vi "(SubVI)I2C_Log.vi"(5 "Data Size":T2, 7 "R/W":T1, 8 "error in (no error)":errorcluster caption="에러 입력(에러 없음)", 9 "Data":u16 format="%.0x", 10 "Address":u16 format="%.0x", 11 "Log Ref":refnum<vi>) -> (0 "error out":errorcluster caption="에러 출력", 3 "Log":string)   [LabVIEW 2020]
uses:
  Controls/(Ctrl)I2C_Data Size.ctl
  Controls/(Ctrl)I2C_RW.ctl
panel:
  # "(SubVI)I2C_Log.vi By hspark\n\nDescription : I2C 통신 결과 Log 문자열을 생성하고 Log 문자열 인디케이터 참조를 연결한 경우 Log를 업데이트 하는VI\n\nInput : \n1. Log Ref : 업데이트할 Log 문자열 인디케이터의 참조. 입력하지 않는 경우 Log 문자열만 출력하고, 인디케이터 업데이트는 무시됨\n2. Address : 생성할 Log의 Address 부분\n3. Data : 생성할 Log의 Data 부분\n4. R/W : Read/Write 구분\n5. Data Size : 생성할 Log의 비트 크기\n\nOutput : \n1. Log : 생성된 Log 문자열 출력\n\nLabVIEW Version : 2020 SP1 이상\n\nNote : 에러 발생 시 에러 종류를 Log로 출력함. \n\nUpdate : 2021.10.06"
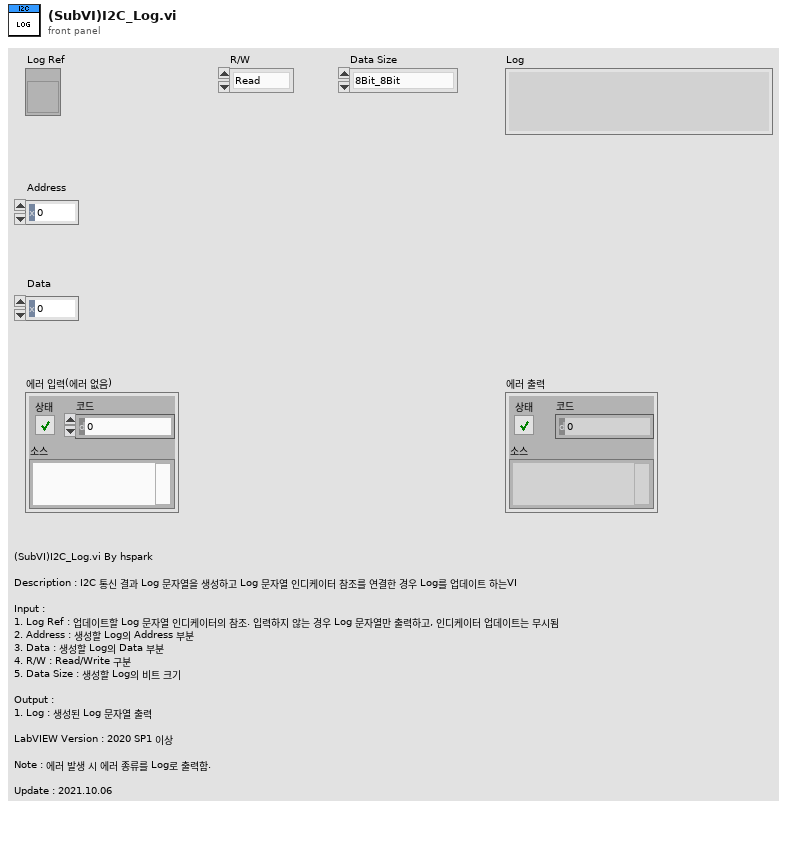
[diagram p1: front panel]
types:
  T1 = typedef "(Ctrl)I2C_RW.ctl" = enum16{"Read", "Write"}
  T2 = typedef "(Ctrl)I2C_Data Size.ctl" = enum16{"8Bit_8Bit", "16Bit_16Bit", "16Bit_8Bit"}
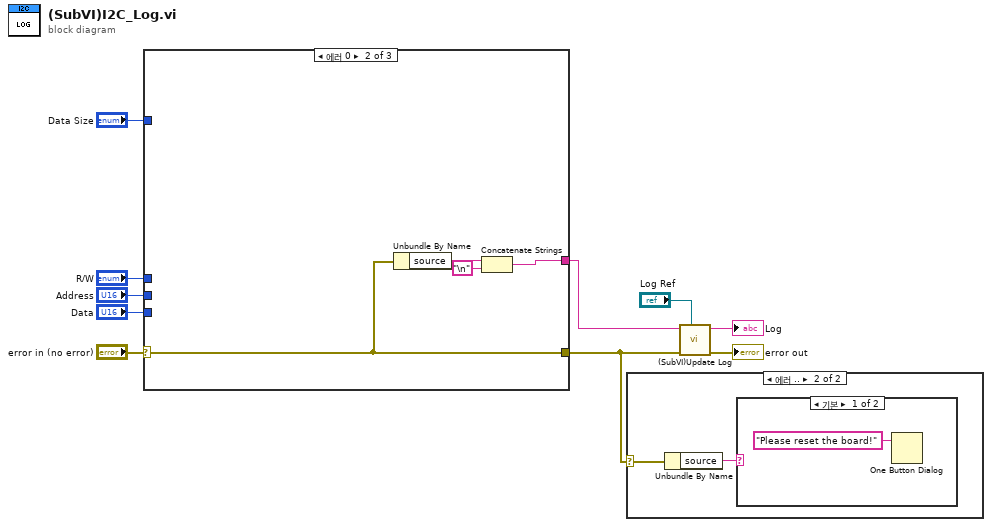
[diagram p0: block diagram]
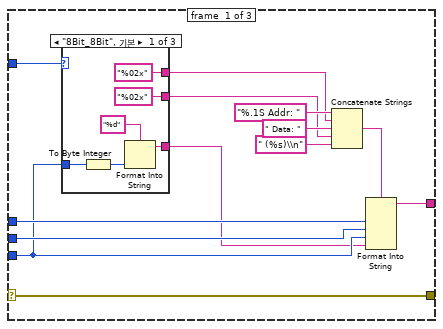
[diagram p4: hidden frame]
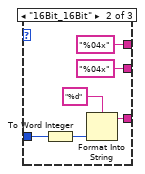
[diagram p5: hidden frame]
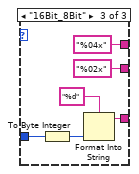
[diagram p6: hidden frame]
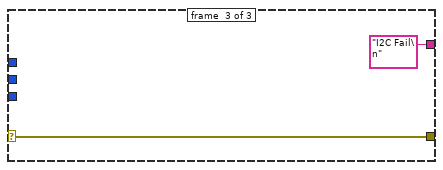
[diagram p7: hidden frame]
diagram:
  n1 = case shown="에러 0" "error in (no error)" {
    selector: "error in (no error)" -> [w13 w42 w47]
    tunnel: "R/W" -> [w23 _ _]
    tunnel: [w22 w44 "I2C Fail\n"] -> w4
    tunnel: "Address" -> [w21 _ _]
    tunnel: "Data" -> [w12 _ _]
    tunnel: "Data Size" -> [w17 _ _]
    tunnel: [w13 w42 w47] -> w1
    frame #0 {
      n2 = case shown="\"8Bit_8Bit\", 기본" w17 {
        tunnel: ["%02x" "%04x" "%04x"] -> w16
        tunnel: ["%02x" "%04x" "%02x"] -> w15
        tunnel: w12 -> [w27 w31 w38]
        tunnel: [w24 w30 w36] -> w11
        frame "8Bit_8Bit", Default {
          n3 = To Byte Integer(number=w27) -> (8bit integer=w26:i8)
          n4 = Format Into String(format string="%d" ("포맷 문자열"), w26) -> (resulting string=w24:string)  [unwired: 2 in, 1 out]
        }
        frame "16Bit_16Bit" {
          n5 = To Word Integer(number=w31) -> (16bit integer=w33:i16)
          n6 = Format Into String(format string="%d" ("포맷 문자열"), w33) -> (resulting string=w30:string)  [unwired: 2 in, 1 out]
        }
        frame "16Bit_8Bit" {
          n7 = To Byte Integer(number=w38) -> (8bit integer=w37:i8)
          n8 = Format Into String(format string="%d" ("포맷 문자열"), w37) -> (resulting string=w36:string)  [unwired: 2 in, 1 out]
        }
      }
      n9 = Concatenate Strings("%.1S Addr: " ("문자열"), w16, " Data: " ("문자열"), w15, " (%s)\\n" ("문자열")) -> (w14:string)
      n10 = Format Into String(format string=w14, w23, w21, w12, w11) -> (resulting string=w22:string)  [unwired: 2 in, 1 out]
    }
    frame #1 {
      n11 = Unbundle By Name(w42) -> ("source"=w45:string)
      n12 = Concatenate Strings(w45, "\n") -> (w44:string)
    }
    frame #2 {
    }
  }
  n13 = case shown="에러 .." w1 {
    selector: w1 -> [_ w49]
    frame No Error {
    }
    frame Error {
      n14 = Unbundle By Name(w49) -> ("source"=w48:string)
      n15 = case shown="기본" w48 {
        frame Default {
          n16 = One Button Dialog(message="Please reset the board!" ("메시지")) -> ()  [unwired: 1 in, 1 out]
        }
        frame "No Ack" {
        }
      }
    }
  }
  n17 = call "(SubVI)Update Log.vi"("Log Ref"="Log Ref", "error in (no error)"=w1, "Log"=w4) -> ("error out"=→"error out":errorcluster, "Log out"=→"Log":string)  [unwired: 7 in]
